vi "CtoF.vi"() -> ()   [LabVIEW 2019]
panel:
  in  "stop":bool
  out "TempF":dbl(slide) scale=0.0..300.0
  in  "TempC":dbl(slide) scale=0.0..100.0
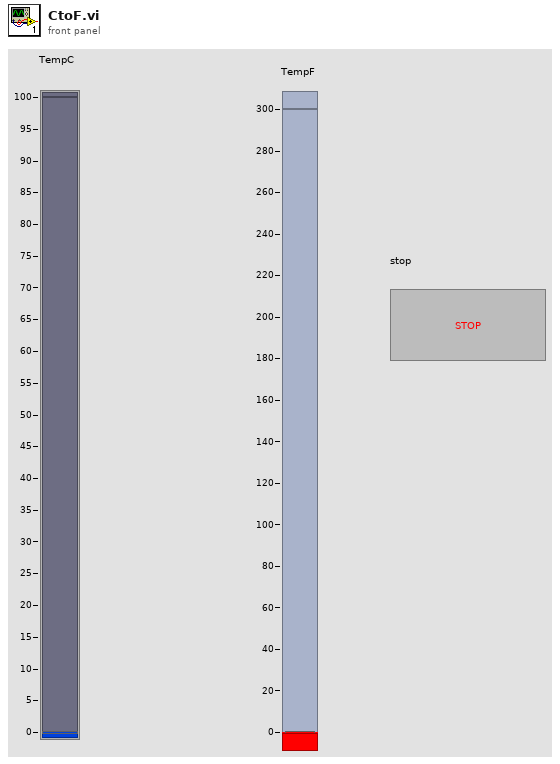
[diagram p1: front panel]
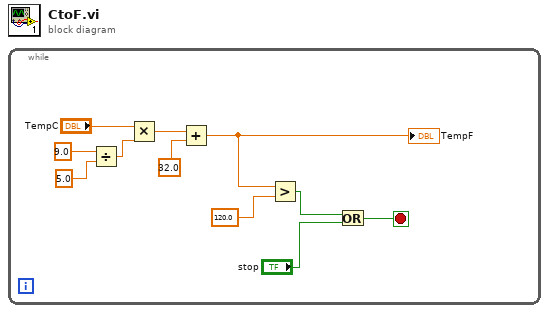
[diagram p0: block diagram]
diagram:
  n1 = while {
    stop <- w1 stop-if-true
    n2 = Divide(x=9.0, y=5.0) -> (x/y=w10:dbl)
    n3 = Multiply(x="TempC", y=w10) -> (x*y=w7:dbl)
    n4 = Add(x=w7, y=32.0) -> (x+y=w5:dbl)
    "TempF" <- w5
    n5 = Greater?(x=w5, y=120.0) -> (0:w3:bool)
    n6 = Or(x=w3, y="stop") -> (x .or. y?=w1:bool)
  }
